vi "Create Item Configurations.vi"(8 "error in (no error)":errorcluster, 11 "Controls References":refnum<vi>[](array[refnum])) -> (0 "error out":errorcluster, 3 "Item Configurations":refnum<class "Item Configuration.lvclass">[](array[class]))   [LabVIEW 2013, in "File IO.lvlib"]
uses:
  File IO.lvlib
  Item Configuration/Item Configuration/Item Configuration.lvclass
  Item Configuration/String Item Configuration/String Item Configuration.lvclass
  Item Configuration/Ring Item Configuration/Ring Item Configuration.lvclass
  Item Configuration/Timestamp Item Configuration/Timestamp Item Configuration.lvclass
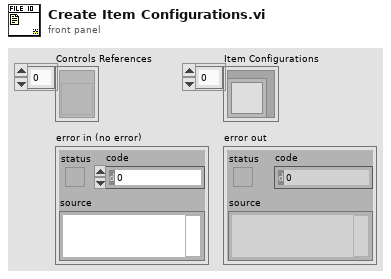
[diagram p1: front panel]
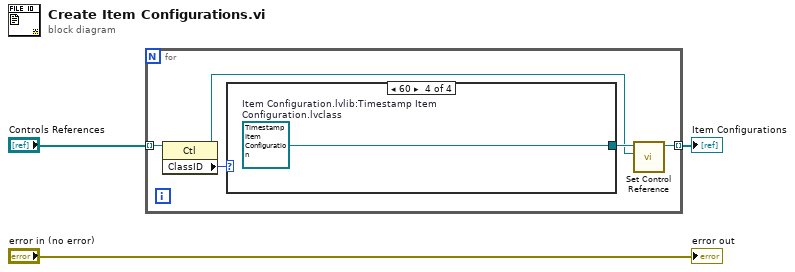
[diagram p0: block diagram]
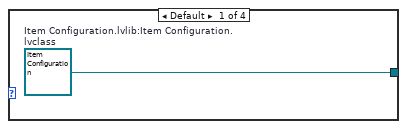
[diagram p2: hidden frame]
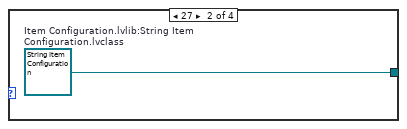
[diagram p3: hidden frame]
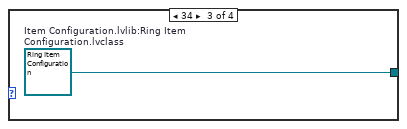
[diagram p4: hidden frame]
diagram:
  n1 = for {
    tunnel: "Controls References" -> [w8] mode=indexing
    tunnel: [w5] -> w1 mode=indexing
    n2 = property class="Ctl"(reference=w8) -> (reference out=w4:refnum<vi>, "ClassID"=w7:u32)  [unwired: 1 in, 1 out]
    n3 = case shown="60" w7 {
      tunnel: [w9 w10 w11 w12] -> w6
      frame Default {
        w9 = refnum<class "Item Configuration.lvclass"> refnum  # Item Configuration.lvlib:Item Configuration.lvclass
      }
      frame 27 {
        w10 = refnum<class "String Item Configuration.lvclass"> refnum  # Item Configuration.lvlib:String Item Configuration.lvclass
      }
      frame 34 {
        w11 = refnum<class "Ring Item Configuration.lvclass"> refnum  # Item Configuration.lvlib:Ring Item Configuration.lvclass
      }
      frame 60 {
        w12 = refnum<class "Timestamp Item Configuration.lvclass"> refnum  # Item Configuration.lvlib:Timestamp Item Configuration.lvclass
      }
    }
    n4 = call-dynamic "Set Control Reference.vi"("Control Reference"=w4, "Item Configuration in"=w6) -> ("Item Configuration out"=w5:refnum<class "Item Configuration.lvclass">)  [unwired: 8 in, 1 out]
  }
  "Item Configurations" <- w1
  "error out" <- "error in (no error)"
